vi "Run Service.vi"() -> ()   [LabVIEW 2021, in "NI DAQmx_server.lvlib"]
uses:
  NI DAQmx_server.lvlib
  <vilib>/gRPC/Generated APIs/ni/measurementlink/discovery/v1/RPC Messages/ni_measurementlink_discovery_v1_RegisterServiceRequest.ctl
  <vilib>/gRPC/Generated APIs/ni/measurementlink/discovery/v1/RPC Messages/ni_measurementlink_discovery_v1_ServiceDescriptor.ctl
  <vilib>/gRPC/Generated APIs/ni/measurementlink/discovery/v1/RPC Messages/ni_measurementlink_discovery_v1_ServiceDescriptor_AnnotationsEntry.ctl
  <vilib>/gRPC/Generated APIs/ni/measurementlink/discovery/v1/RPC Messages/ni_measurementlink_discovery_v1_ServiceLocation.ctl
  RPC Service/NiDAQmx/NiDAQmx.lvclass
  C:/Program Files/National Instruments/LabVIEW 2021/vi.lib/gRPC/LabVIEW gRPC Servicer/ServiceBase/ServiceBase.lvclass
  <vilib>/gRPC/LabVIEW gRPC Servicer/Servicer/Servicer.lvclass/Servicer.ctl
  <vilib>/gRPC/LabVIEW gRPC Servicer/Servicer/Servicer.lvclass
  <vilib>/Plug-In SDKs/Clients/Discovery V1/NI Discovery V1 Client.lvlib
  <vilib>/gRPC/Generated APIs/ni/measurementlink/discovery/v1/ni.measurementlink.discovery.v1.api.lvlib
panel:
  out "error out":errorcluster
  out "Listening Port":i32
  in  "Stop":bool
  in  "Server Certificate File (.crt)":path
  in  "Server Key File (.key)":path
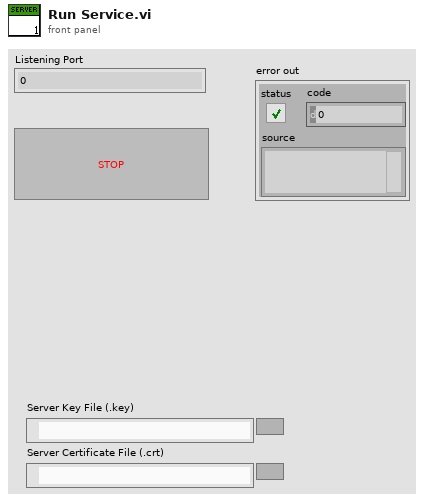
[diagram p1: front panel]
types:
  T1 = typedef "ni.measurementlink.discovery.v1.api.lvlib/ni_measurementlink_discovery_v1_RegisterServiceRequest.ctl" = cluster{"service_description":T2, "location":T4}
  T2 = typedef "ni.measurementlink.discovery.v1.api.lvlib/ni_measurementlink_discovery_v1_ServiceDescriptor.ctl" = cluster{"display_name":string, "description_url":string, "provided_interfaces":string[], "service_class":string, "annotations":T3[], "versions":string[]}
  T3 = typedef "ni.measurementlink.discovery.v1.api.lvlib/ni_measurementlink_discovery_v1_ServiceDescriptor_AnnotationsEntry.ctl" = cluster{"key":string, "value":string}
  T4 = typedef "ni.measurementlink.discovery.v1.api.lvlib/ni_measurementlink_discovery_v1_ServiceLocation.ctl" = cluster{"location":string, "insecure_port":string, "ssl_authenticated_port":string}
  T5 = enum32{"Invalid", "Standard", "Closed", "Hidden", "Minimized", "Maximized"}
  T6 = typedef "grpc-lvsupport-release.lvlib/grpcId.ctl" = u64
  T7 = typedef "ni.measurementlink.discovery.v1.api.lvlib/ni_measurementlink_discovery_v1_RegisterServiceResponse.ctl" = cluster{"registration_id":string}
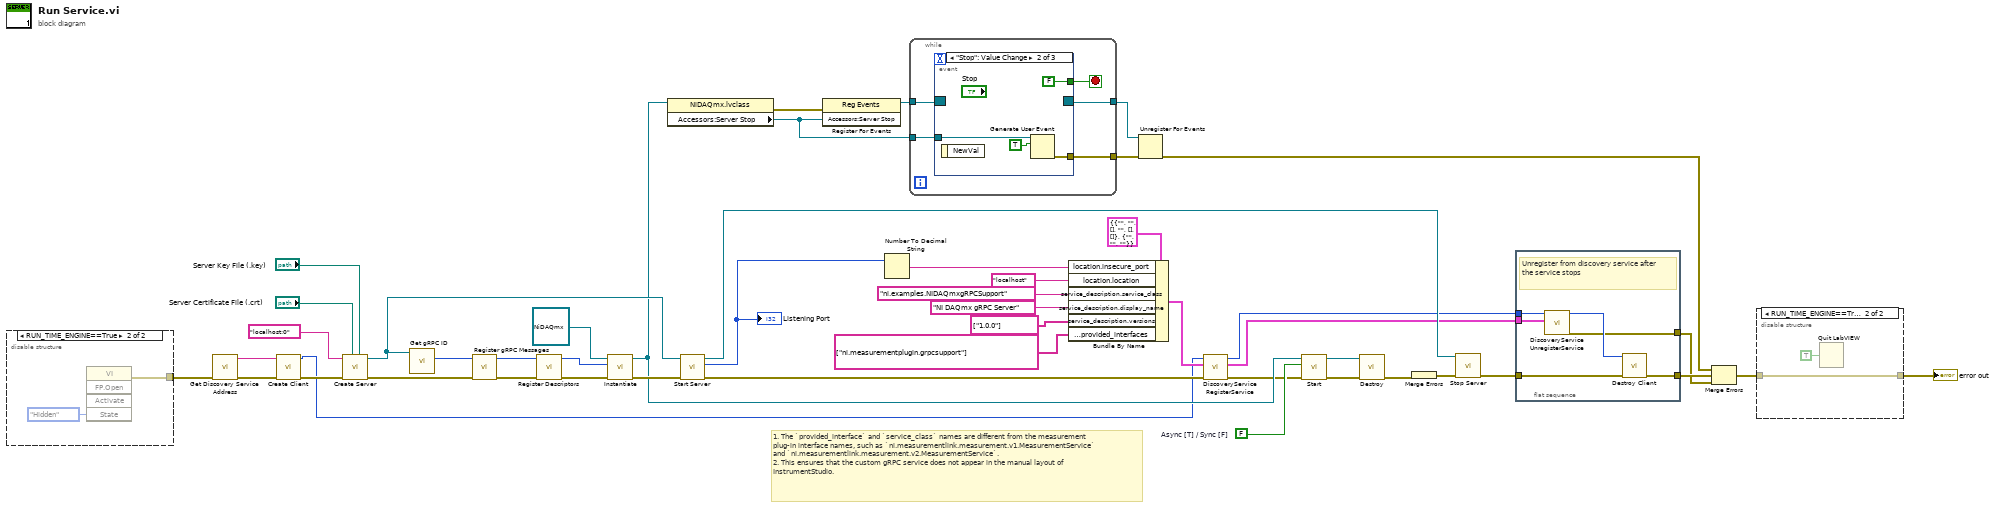
[diagram p0: block diagram]
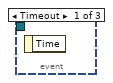
[diagram p3: hidden frame]
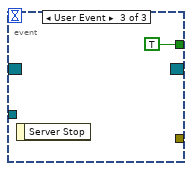
[diagram p4: hidden frame]
diagram:
  w30 = FALSE  # Async [T] / Sync [F]
  # "1. The `provided_interface` and `service_class` names are different from the measurement plug-in interface names, such as `ni.measurementlink.measurement.v1.MeasurementService` and `ni.measurementlink.measurement.v2.MeasurementService`.\n2. This ensures that the custom gRPC service does not appear in the manual layout of InstrumentStudio."
  n1 = disable-structure shown="RUN_TIME_ENGINE==True" {
    disable-tunnel: [_ w49] -> w25
    frame condition #0 (active) {
    }
    frame condition #1 {
      n2 = invoke class="VI" method="FP.Open"("State"=T5."Hidden") -> (error out=w49:errorcluster)  [unwired: 4 in, 4 out]
    }
  }
  n3 = call <vilib>:"Get Discovery Service Address.vi"("error in"=w25) -> ("error out"=w24:errorcluster, "address"=w23:string)  [unwired: 9 in]
  n4 = call <vilib>:"Create Client.vi"("error in"=w24, "address"=w23) -> ("error out"=w22:errorcluster, "gRPC ID Out"=w9:T6)  [unwired: 8 in]
  n5 = call <vilib>:"Create Server.vi"("Server Key File (.key)"="Server Key File (.key)", "Server Certificate File (.crt)"="Server Certificate File (.crt)", "error in"=w22, "Server Address"="localhost:0") -> ("error out"=w35:errorcluster, "gRPC Server out"=w42:refnum<class "Servicer.lvclass">)  [unwired: 6 in]
  n6 = call <vilib>:"Get gRPC ID.vi"("OOP Server in"=w42) -> ("gRPC ID"=w36:T6)  [unwired: 9 in, 1 out]
  n7 = call "Register gRPC Messages.vi"("error in (no error)"=w35, "gRPC ID"=w36) -> ("error out"=w27:errorcluster, "gRPC ID Out"=w26:T6)  [unwired: 8 in]
  n8 = call "Register Descriptors.vi"("error in (no error)"=w27, "gRPC ID"=w26) -> ("error out"=w34:errorcluster, "gRPC ID Out"=w33:T6)  [unwired: 8 in]
  n9 = call-dynamic "Instantiate.vi"("error in"=w34, "gRPCid"=w33, "iService"=refnum<class "NiDAQmx.lvclass"> refnum ("NI DAQmx_server.lvlib:NiDAQmx.lvclass")) -> ("error out"=w40:errorcluster, "iService"=w29:refnum<class "NiDAQmx.lvclass">)  [unwired: 7 in]
  n10 = property class="NiDAQmx.lvclass"(reference=w29) -> (error out=w41:errorcluster, "Accessors:Server Stop"=w28:refnum<user-event>)  [unwired: 1 in, 1 out]
  n11 = call <vilib>:"Start Server.vi"("error in"=w40, "gRPC Server in"=w42) -> ("error out"=w12:errorcluster, "Listening Port"=w13:i32, "gRPC Server out"=w48:refnum<class "Servicer.lvclass">)  [unwired: 7 in]
  "Listening Port" <- w13
  n12 = register-events(error in=w41, w28) -> (reference out=w44:refnum<event-registration>)  [unwired: 1 in, 1 out]
  n13 = Number To Decimal String(number=w13) -> (decimal integer string=w19:string)  [unwired: 1 in]
  n14 = while {
    tunnel: w44 -> [w55]
    tunnel: [w53] -> w43
    tunnel: [w51] -> w37
    tunnel: w28 -> [w52]
    stop <- w54 stop-if-true
    n15 = event shown="[1] \"Stop\": Value Change" {
      selector: w55 -> [_ _ _]
      dyn-events: [_ _ _] -> w53
      timeout: _ -> [_ _ _]
      tunnel: [_ FALSE TRUE] -> w54
      tunnel: w52 -> [_ w58 _]
      tunnel: [_ w56 _] -> w51
      event Timeout {
        n16 = event-data() -> ()  [unwired: 1 in, 1 out]
      }
      event "Stop": Value Change {
        n17 = event-data() -> ()  [unwired: 1 in, 1 out]
        n18 = Generate User Event(user event=w58, event data cluster=TRUE ("event data")) -> (error out=w56:errorcluster)  [unwired: 2 in, 1 out]
      }
      event User Event {
        n19 = event-data() -> ()  [unwired: 1 in, 1 out]
      }
    }
  }
  n20 = Bundle By Name(cluster=T1 {"service_description"={"display_name"="", "description_url"="", "provided_interfaces"=[], "service_class"="", "annotations"=[], "versions"=[]}, "location"={"location"="", "insecure_port"="", "ssl_authenticated_port"=""}} ("Request Data"), "location.insecure_port"=w19, "location.location"="localhost", "service_description.service_class"="ni.examples.NIDAQmxgRPCSupport", "service_description.display_name"="NI DAQmx gRPC Server", "service_description.versions"=string[] ["1.0.0"], "service_description.provided_interfaces"=string[] ["ni.measurementplugin.grpcsupport"]) -> (w10:T1)
  n21 = Unregister For Events(event registration refnum=w43, error in=w37) -> (error out=w3:errorcluster)
  n22 = call <vilib>:"DiscoveryService RegisterService.vi"("error in"=w12, "Request Data"=w10, "gRPC ID"=w9) -> ("error out"=w11:errorcluster, "Response Data"=w6:T7, "gRPC ID out"=w7:T6)  [unwired: 6 in]
  n23 = call-dynamic "Start.vi"("error in"=w11, "ASync [T]"=w30, "iService in"=w29) -> ("error out"=w32:errorcluster, "iService out"=w31:refnum<class "NiDAQmx.lvclass">)  [unwired: 7 in]
  n24 = call-dynamic "Destroy.vi"("error in (no error)"=w32, "SignalGeneratorService in"=w31) -> ("error out"=w39:errorcluster)  [unwired: 8 in, 1 out]
  n25 = Merge Errors(w39) -> (w38:errorcluster)
  n26 = call <vilib>:"Stop Server.vi"("error in"=w38, "gRPC Server in"=w48) -> ("error out"=w8:errorcluster)  [unwired: 9 in]
  n27 = flat-sequence {
    tunnel: w7 -> [w66]
    tunnel: w6 -> [w65]
    tunnel: [w64] -> w5
    tunnel: w8 -> [w61]
    tunnel: [w62] -> w4
    frame #0 {
      # "Unregister from discovery service after the service stops"
      n28 = call <vilib>:"DiscoveryService UnregisterService.vi"("Request Data"=w65, "gRPC ID"=w66) -> ("error out"=w62:errorcluster, "gRPC ID out"=w63:T6)  [unwired: 7 in, 1 out]
      n29 = call <vilib>:"Destroy Client.vi"("error in"=w61, "gRPC ID"=w63) -> ("error out"=w64:errorcluster)  [unwired: 9 in]
    }
  }
  n30 = Merge Errors(w3, w5, w4) -> (w2:errorcluster)
  n31 = disable-structure shown="RUN_TIME_ENGINE==True" {
    disable-tunnel: w2 -> [w67 w68]
    disable-tunnel: [w67 w68] -> w1
    frame condition #0 (active) {
    }
    frame condition #1 {
      n32 = Quit LabVIEW(quit? (T)=TRUE) -> ()
    }
  }
  "error out" <- w1
